vi "ClearNoise analisis kill.vi"() -> ()   [LabVIEW 2015, in "VIPM2.lvlib"]
uses:
  VIPM2.lvlib
panel:
  out "Stop Acquisition?":bool
  in  "ACQ full DATA file path":path caption="File path"
  in  "Log it":i32
  in  "Addresses Cluster":T1={"ENA1"=FALSE, "IP address 1"="172.16.14.22", "ENA2"=FALSE, "IP address 2"="172.16.14.23"}
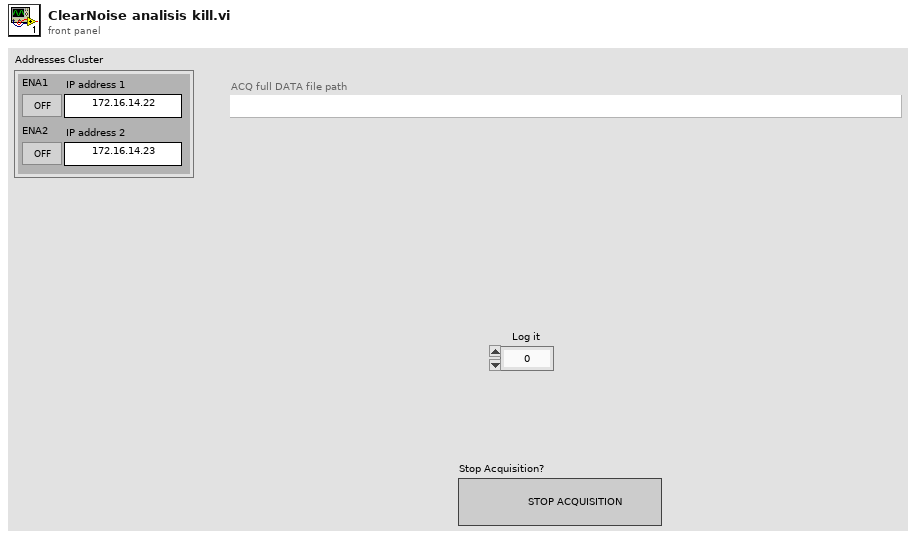
[diagram p1: front panel]
types:
  T1 = cluster{"ENA1":bool, "IP address 1":string, "ENA2":bool, "IP address 2":string}
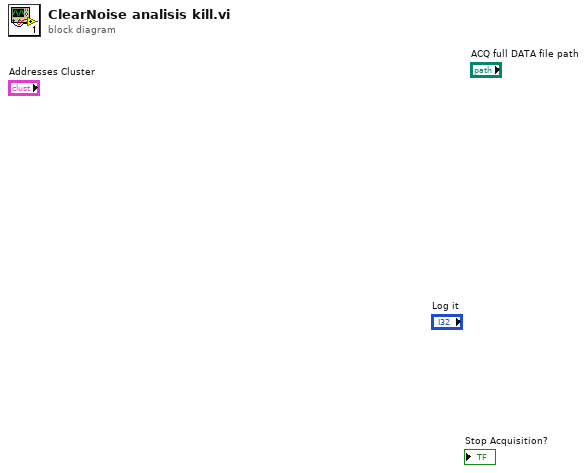
[diagram p0: block diagram]
diagram:
